vi "get object list.vi"() -> (16 "Objects":string[](array[string]))   [LabVIEW 2014, in "PTUtils.lvlib"]
uses:
  PTUtils.lvlib
  CSCore/CSSystem/CSSystemLib/CSSystemLib.lvlib
  CSlibraries-extern/DimLVEvent/LVDimInterface/LVDimInterface.lvlib
  CSCore/CSSystem/CoreLib/CoreLib.lvlib
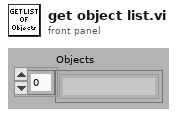
[diagram p1: front panel]
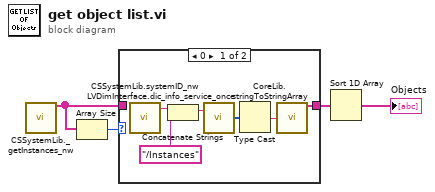
[diagram p0: block diagram]
diagram:
  n1 = call "CSSystemLib._getInstances_nw.vi"() -> ("i list"=w2:string[])  [unwired: 18 in, 1 out]
  n2 = Array Size(array=w2) -> (size(s)=w4:i32)
  n3 = case shown="0" w4 {
    tunnel: [w8 w11] -> w3
    tunnel: w2 -> [_ w11]
    frame 0 {
      n4 = call "CSSystemLib.systemID_nw.vi"() -> ("systemID out"=w10:string)  [unwired: 18 in, 1 out]
      n5 = Concatenate Strings(w10, "/Instances" ("string")) -> (w9:string)
      n6 = call "LVDimInterface.dic_info_service_once.vi"("serviceName"=w9) -> ("data"=w7:i8[])  [unwired: 15 in, 3 out]
      n7 = Type Cast(x=w7) -> (*(type *) &x=w6:string)  [unwired: 1 in]
      n8 = call "CoreLib.stringToStringArray.vi"("String"=w6) -> ("Array"=w8:string[])
    }
    frame 1, Default {
    }
  }
  n9 = Sort 1D Array(array=w3) -> (sorted array=→"Objects":string[])
